vi "Explode String.vi"(7 "Delimiter (comma)":string=",", 11 "String":string) -> (3 "Array":string[](array[string]))   [LabVIEW 2012, in "nmea.lvlib" / "NMEA Message.lvclass"]
uses:
  NMEA Message.lvclass
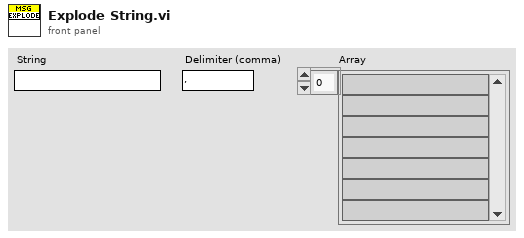
[diagram p1: front panel]
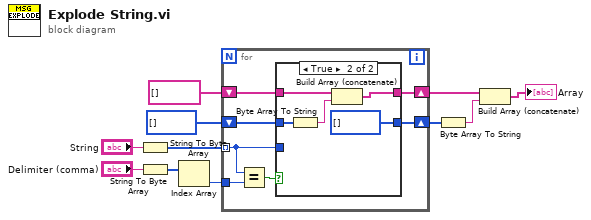
[diagram p0: block diagram]
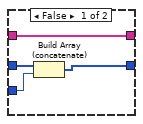
[diagram p2: hidden frame]
diagram:
  n1 = String To Byte Array(string="String") -> (unsigned byte array=w7:u8[])
  n2 = String To Byte Array(string="Delimiter (comma)") -> (unsigned byte array=w9:u8[])
  n3 = Index Array(array=w9) -> (element=w8:u8)  [unwired: 1 in]
  n4 = for {
    tunnel: w8 -> [w18]
    tunnel: w7 -> [w15] mode=indexing
    shift-right: [w14] -> w4
    shift-left: u8[] [] ("unsigned byte array") -> [w17]
    shift-right: [w12] -> w3
    shift-left: string[] [] ("Array") -> [w13]
    n5 = Equal?(x=w15, y=w18) -> (x = y?=w16:bool)
    n6 = case shown="True" w16 {
      tunnel: w17 -> [w22 w27]
      tunnel: w15 -> [w21 _]
      tunnel: [w20 u8[] []] -> w14
      tunnel: w13 -> [w19 w26]
      tunnel: [w19 w24] -> w12
      frame False {
        n7 = Build Array (concatenate)(w22, w21) -> (w20:u8[])
      }
      frame True {
        n8 = Byte Array To String(unsigned byte array=w27) -> (string=w25:string)
        n9 = Build Array (concatenate)(w26, w25) -> (w24:string[])
      }
    }
  }
  n10 = Byte Array To String(unsigned byte array=w4) -> (string=w1:string)
  n11 = Build Array (concatenate)(w3, w1) -> (→"Array":string[])
